vi "demo - niScope EX Simulated Acquisition.vi"() -> ()   [LabVIEW 2024]
doc: "#vi_description \nSimulates a 2 ch digitizer and plots the graph. This is an NI example from NI-SCOPE that has been modifed.\nThetic Engineering Ltd."
uses:
  <instrlib>/niScope/Configure/Trigger/niScope Configure Trigger Edge.vi
  <instrlib>/niScope/Configure/Trigger/niScope Configure Trigger Digital.vi
  <instrlib>/niScope/Configure/Trigger/niScope Configure Trigger Immediate.vi
  <instrlib>/niScope/Acquire/niScope Multi Read Cluster.vi
panel:
  out "Option String":string
  in  "Simulate":bool
  in  "Stop":bool caption="stop"
  in  "Model":u16(ring)=3 items=["NI-5102", "NI-5105", "NI-5112", "NI-5114", "NI-5122", "NI-5124", "NI-5132", "NI-5133", "NI-5142", "NI-5152", "NI-5153", "NI-5154", "NI-5160 (2CH)", "NI-5160 (4CH)", "NI-5162 (2CH)", "NI-5162 (4CH)", "NI-5170R (4CH)", "NI-5170R (8CH)", "NI-5171R (8CH)", "NI-5185", "NI-5186", "NI-5620", "NI-5621", "NI-5622", "NI-5911", "NI-5922"]
  in  "Board Type":u16(ring)=1 items=["PCI", "PXI", "PXIe", "USB", "AT", "PCMCIA"]
  in  "Channel(s)":string="0,1"
  in  "Resource Name":refnum<k15>="Dev1" caption="Resource Name(s)"
  out "Waveform Graph":T1(graph)
  in  "Number Of Records":i32=1 step=1
  out "Actual Sample Rate":dbl format="%#.3p"
  out "Actual Record Length":i32=1000
  in  "Min. Record Length":i32=1000
  in  "Min. Sample Rate":dbl=1000000.0 step=1000000.0 format="%#.3p"
  in  "Max. Input Frequency (Hz)":dbl caption="Max. Input\nFrequency (Hz)" format="%.2f"
  in  "Input Impedance":u32(ring) items=["1 mega ohm", "75 ohms", "50 ohms"]
  in  "Vertical Coupling":i32(ring) items=["AC", "DC", "Ground"]
  in  "Vertical Noise \n(% Range)":dbl=4.0 format="%.2f"
  in  "Vertical Range (V)":dbl=5.0 format="%.2f"
  in  "Trigger Source":string(combo)="0"
  in  "Trigger Level (V)":dbl format="%.2f"
  in  "Ref Position":dbl=50.0 format="%.1f"
  in  "Trigger Slope":i32(ring) items=["Positive", "Negative"]
  in  "Trigger Type":u16(ring)=2 items=["Edge", "Digital", "Immediate"]
  # "General"
  # "Horizontal"
  # "Channel"
  # "Vertical"
  # "Trigger"
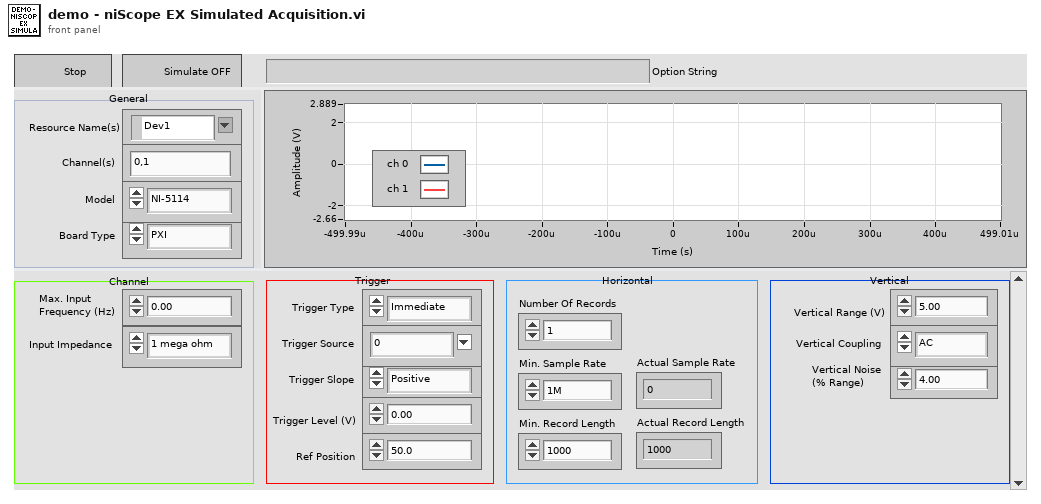
[diagram p1: front panel]
types:
  T1 = cluster{"relativeInitialX":dbl, "xIncrement":dbl, "wfm":dbl[]}[]
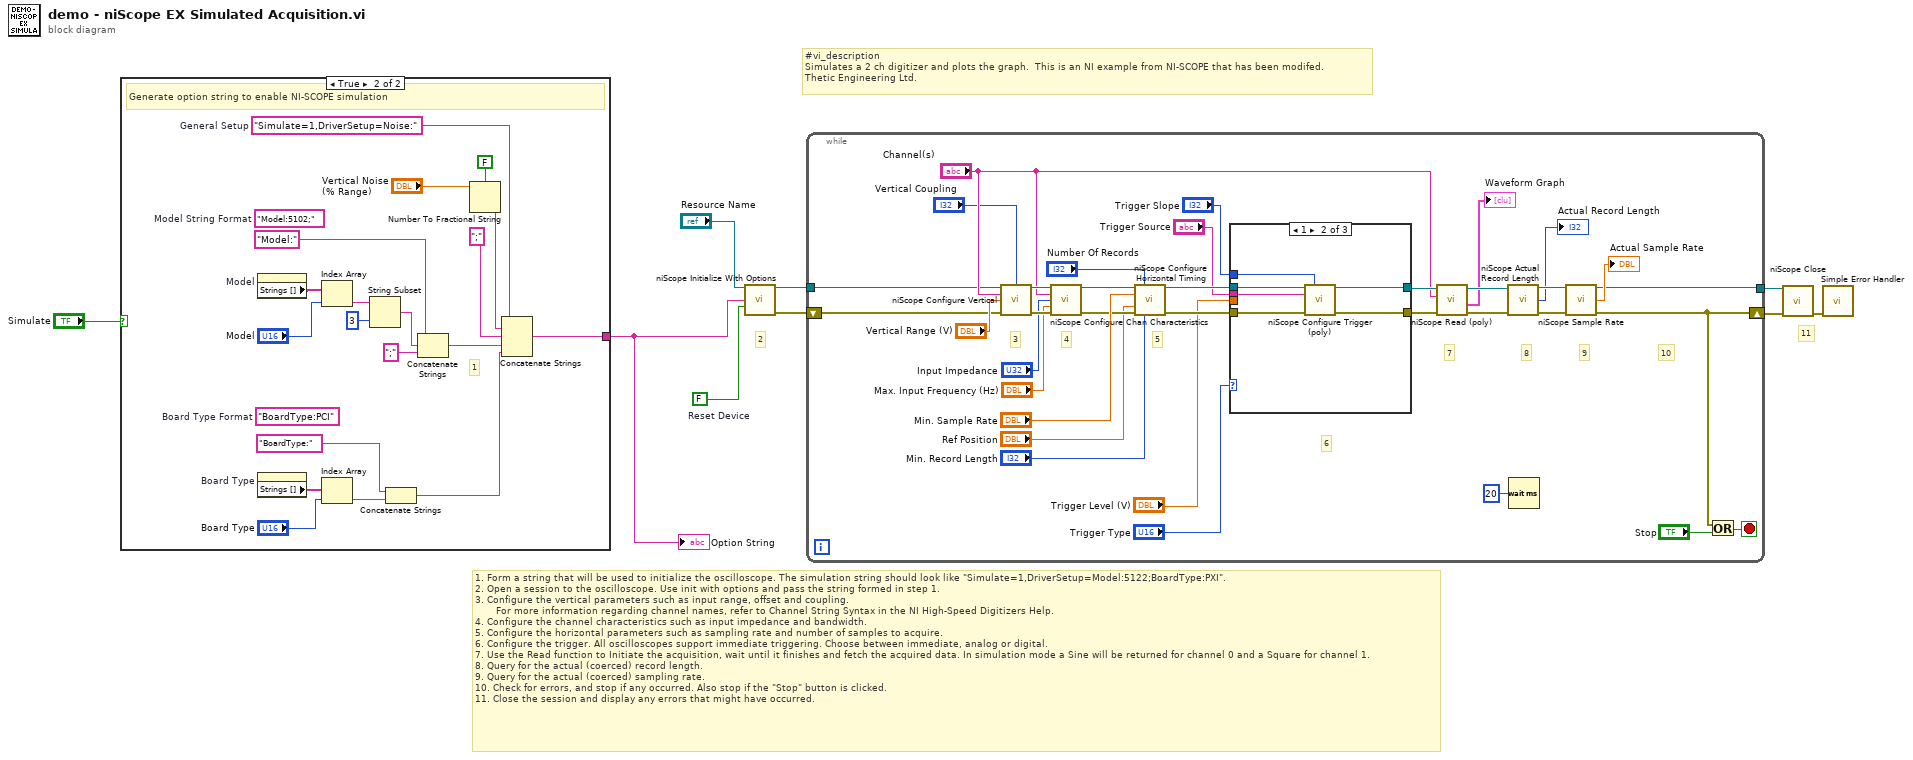
[diagram p0: block diagram]
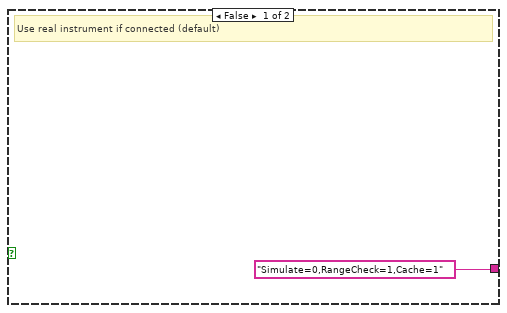
[diagram p2: hidden frame]
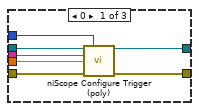
[diagram p3: hidden frame]
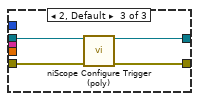
[diagram p4: hidden frame]
diagram:
  w8 = FALSE  # Reset Device
  # "#vi_description \nSimulates a 2 ch digitizer and plots the graph.  This is an NI example from NI-SCOPE that has been modifed.\nThetic Engineering Ltd."
  # "11"
  # "1. Form a string that will be used to initialize the oscilloscope. The simulation string should look like \"Simulate=1,DriverSetup=Model:5122;BoardType:PXI\".\n2. Open a session to the oscilloscope. Use init with options and pass the string formed in step 1.\n3. Configure the vertical parameters such as input range, offset and coupling.\n       For more information regarding channel names, refer to Channel String Syntax in the NI High-Speed Digitizers Help.\n4. Configure the channel characteristics such as input impedance and bandwidth.\n5. Configure the horizontal parameters such as sampling rate and number of samples to acquire.\n6. Configure the trigger. All oscilloscopes support immediate triggering. Choose between immediate, analog or digital.\n7. Use the Read function to Initiate the acquisition, wait until it finishes and fetch the acquired data. In simulation mode a Sine will be returned for channel 0 and a Square for channel 1.\n8. Query for the actual (coerced) record length.\n9. Query for the actual (coerced) sampling rate.\n10. Check for errors, and stop if any occurred. Also stop if the \"Stop\" button is clicked.\n11. Close the session and display any errors that might have occurred."
  # "2"
  n1 = case shown="True" "Simulate" {
    tunnel: ["Simulate=0,RangeCheck=1,Cache=1" ("option string") w25] -> w1
    frame False {
      # "Use real instrument if connected (default)"
    }
    frame True {
      (unwired) "BoardType:PCI"  # Board Type Format
      (unwired) "Model:5102;"  # Model String Format
      w28 = "Simulate=1,DriverSetup=Noise:"  # General Setup
      # "1"
      # "Generate option string to enable NI-SCOPE simulation"
      n2 = property on="Model" class="Ring (strict)"() -> ("Strings []"=w24:string[])  [unwired: 2 in, 2 out]
      n3 = property on="Board Type" class="Ring (strict)"() -> ("Strings []"=w16:string[])  [unwired: 2 in, 2 out]
      n4 = Index Array(array=w24, index="Model") -> (element=w22:string)
      n5 = Index Array(array=w16, index="Board Type") -> (element=w14:string)
      n6 = String Subset(string=w22, offset (0)=3 ("Offset (0)")) -> (substring=w19:string)  [unwired: 1 out]
      n7 = Concatenate Strings("BoardType:" ("Board Type Format"), w14) -> (w12:string)
      n8 = Concatenate Strings("Model:" ("String"), w19, ";" ("String")) -> (w20:string)
      n9 = Number To Fractional String(use system decimal point (T)=FALSE ("Use System Decimal Point (T)"), number="Vertical Noise \n(% Range)") -> (F-format string=w27:string)  [unwired: 2 out]
      n10 = Concatenate Strings(w28, w27, ";", w20, w12) -> (w25:string)
    }
  }
  "Option String" <- w1
  n11 = call <instrlib>:"niScope Initialize With Options.vi"("resource name"="Resource Name", "option string"=w1, "reset device"=w8) -> ("instrument handle"=w6:refnum<k15>, "error out"=w5:errorcluster)  [unwired: 2 in, 9 out]
  n12 = while {
    tunnel: w6 -> [w32]
    tunnel: [w38] -> w4
    shift-right: [w37] -> w3
    shift-left: w5 -> [w31]
    stop <- w39 stop-if-true
    # "10"
    # "9"
    # "8"
    # "6"
    # "7"
    # "5"
    # "4"
    # "3"
    n13 = call <instrlib>:"niScope Configure Vertical.vi"("instrument handle"=w32, "vertical coupling"="Vertical Coupling", "channels"="Channel(s)", "vertical range"="Vertical Range (V)", "error in"=w31) -> ("instrument handle out"=w57:refnum<k15>, "error out"=w56:errorcluster)  [unwired: 3 in, 6 out]
    n14 = call <instrlib>:"niScope Configure Chan Characteristics.vi"("instrument handle"=w57, "channels"="Channel(s)", "input impedance"="Input Impedance", "maximum input frequency"="Max. Input Frequency (Hz)", "error in"=w56) -> ("instrument handle out"=w54:refnum<k15>, "error out"=w55:errorcluster)  [unwired: 9 out]
    n15 = call <instrlib>:"niScope Configure Horizontal Timing.vi"("instrument handle"=w54, "number of records"="Number Of Records", "min sample rate"="Min. Sample Rate", "reference position"="Ref Position", "error in"=w55, "min record length"="Min. Record Length") -> ("instrument handle out"=w50:refnum<k15>, "error out"=w51:errorcluster)  [unwired: 1 in, 7 out]
    n16 = case "Trigger Selection" shown="1" "Trigger Type" {
      tunnel: w51 -> [w71 w77 w81]
      tunnel: [w67 w73 w78] -> w43
      tunnel: w50 -> [w70 w76 w80]
      tunnel: [w68 w74 w79] -> w44
      tunnel: "Trigger Source" -> [w69 w75 _]
      tunnel: "Trigger Level (V)" -> [w66 _ _]
      tunnel: "Trigger Slope" -> [w65 w72 _]
      frame 0 {
        n17 = call-poly <instrlib>:"niScope Configure Trigger (poly).vi"("instrument handle"=w70, "trigger slope"=w65, "trigger source"=w69, "trigger level"=w66, "error in"=w71) -> ("instrument handle out"=w68:refnum<k15>, "error out"=w67:errorcluster)  [unwired: 3 in, 6 out]
      }
      frame 1 {
        n18 = call-poly <instrlib>:"niScope Configure Trigger (poly).vi"("instrument handle"=w76, "trigger slope"=w72, "trigger source"=w75, "error in"=w77) -> ("instrument handle out"=w74:refnum<k15>, "error out"=w73:errorcluster)  [unwired: 2 in, 8 out]
      }
      frame 2, Default {
        n19 = call-poly <instrlib>:"niScope Configure Trigger (poly).vi"("instrument handle"=w80, "error in"=w81) -> ("instrument handle out"=w79:refnum<k15>, "error out"=w78:errorcluster)  [unwired: 12 out]
      }
    }
    n20 = call-poly <instrlib>:"niScope Read (poly).vi"("error in"=w43, "channels"="Channel(s)", "instrument handle"=w44) -> ("error out"=w41:errorcluster, "waveform"=→"Waveform Graph":T1, "instrument handle out"=w42:refnum<k15>)  [unwired: 2 in, 4 out]
    n21 = call <instrlib>:"niScope Actual Record Length.vi"("instrument handle"=w42, "error in"=w41) -> ("instrument handle out"=w61:refnum<k15>, "actual record length"=→"Actual Record Length":i32, "error out"=w60:errorcluster)  [unwired: 11 out]
    n22 = Wait (ms)(milliseconds to wait=u32 20 ("Milliseconds To Wait")) -> ()  [unwired: 1 out]
    n23 = call <instrlib>:"niScope Sample Rate.vi"("instrument handle"=w61, "error in"=w60) -> ("instrument handle out"=w38:refnum<k15>, "actual sample rate"=→"Actual Sample Rate":dbl, "error out"=w37:errorcluster)  [unwired: 11 out]
    n24 = Or(x=w37, y="Stop") -> (x .or. y?=w39:bool)
  }
  n25 = call <instrlib>:"niScope Close.vi"("instrument handle"=w4, "error in"=w3) -> ("error out"=w7:errorcluster)  [unwired: 13 out]
  n26 = call <vilib>:"Simple Error Handler.vi"("error in (no error)"=w7) -> ()  [unwired: 1 in, 8 out]
